vi "PAC-SLI.vi"() -> ()   [LabVIEW 2017]
uses:
  <vilib>/MakerHub/LINX/Private/Type Defs/Peripherals/SPI/SPI Configuration.ctl
  <vilib>/MakerHub/LINX/Private/Type Defs/Peripherals/SPI/SPI Bit Order.ctl
  <vilib>/MakerHub/LINX/Private/Type Defs/Peripherals/SPI/SPI Mode.ctl
  <vilib>/MakerHub/LINX/Public/Peripherals/SPI/SPI CS Config.ctl
  <vilib>/MakerHub/LINX/Private/Type Defs/Peripherals/SPI/SPI CS Logic Level.ctl
  <vilib>/Analysis/Matrix/Datatypes/RealMatrix.ctl
  <vilib>/MakerHub/LINX/Public/Peripherals/PWM/PWM Set Duty Cycle 1 Chan.vi
  <vilib>/MakerHub/LINX/Public/Peripherals/Analog/Analog Read 1 Chan.vi
  <vilib>/MakerHub/LINX/Public/Peripherals/Analog/Analog Read N Chans.vi
  <vilib>/MakerHub/LINX/Private/Local IO/LinxAnalogRead.vi
  <vilib>/MakerHub/LINX/Public/Utilities/Check Channel.vi
  <vilib>/MakerHub/LINX/Public/Utilities/Open Serial.vi
  <vilib>/MakerHub/LINX/Public/Peripherals/PWM/PWM Set Duty Cycle N Chans.vi
  <vilib>/MakerHub/LINX/Private/Utilties/Generate Error.vi
  <vilib>/Analysis/Matrix/Numeric/Conversions/Matrix To Array - RM.vi
  <vilib>/MakerHub/LINX/LMH-LINX.lvlib
  <vilib>/Analysis/Matrix/NI_Matrix.lvlib
panel:
  out "stop 2":bool
  out "Connection Initialized":bool
  out "Debug console":string
  in  "reset":bool
  in  "stop":bool
  out "I/O Device Name":string
  in  "?":T1(tab)
  in  "StayON 6":bool
  in  "StayON 5":bool
  in  "StayON 4":bool
  in  "StayON 3":bool
  in  "StayON 2":bool
  in  "StayON 1":bool
  in  "START Button":bool
  in  "Detector  6":bool
  out "Det 6 status":bool
  in  "Detector  5":bool
  out "Det 5 status":bool
  in  "Detector  4":bool
  out "Det 4 status":bool
  in  "Detector 3":bool
  out "Det 3 status":bool
  in  "Detector 2":bool
  out "Det 2 status":bool
  in  "Detector 1":bool
  out "Det 1 status":bool
  out "Photogate AIN":u8
  out "Stepper PUL DOUT":u8
  out "Stepper DIR DOUT":u8
  out "Stepper ENA DOUT":u8
  out "DigiPAC UART":u8
  out "Thermocouple 1":string
  out "Thermocouple 2":string
  out "Furnace ctrl Channel":u8
  out "Beam gate channel":u8
  in  "Furnace power% set":u8 max=100
  out "Furnace power%":u8
  out "Elapsed Super\nCycle Time (s)":dbl caption="Elapsed Time (s)"
  in  "Supercycle time [s]":dbl
  in  "CS Configuration":T2={"CS Channel"=7, "CS Logic Level"=enum."Active High"}
  in  "SPI Configuration":T4={"Clock Frequency"=1000000, "Bit Order"=enum."LSb First", "SPI Mode"=enum."Mode 0"}
  out "Clock Frequency":u32
  in  "CS Configuration 2":T2={"CS Channel"=7, "CS Logic Level"=enum."Active High"}
  in  "Photogate AIN":u8
  in  "Stepper PUL DOUT":u8
  in  "Stepper DIR DOUT":u8
  in  "Stepper ENA DOUT":u8
  in  "DigiPAC UART":u8
  in  "Furnace ctrl Channel":u8
  in  "Beam gate channel":u8
  in  "Operation|Time":T7
  in  "Serial Port":refnum<visa-resource-name>="COM3"
  # "Check settings before running!"
  # "I/O Channels"
  # "Temperature"
  # "Set      Status"
  # "Furnace power output"
  # "DIN.............."
  # "Digital input"
  # "DOUT.........."
  # "Digital output"
  # "AIN.............."
  # "Analog input"
  # "UART..........."
  # "Serial port"
  # "I/O ports"
  # "Thermocouple SPI settings"
  # "Automation order and timing"
  # "Thermocouple SPI settings required by MAX31855 amplifier:\nCS Logic level.............Active Low\nBit Order......................MSb First\nSPI Mode.....................Mode 0\nClock Frequency........<15000000\n                                      12500 is ok\nMISO/Data port...........50\nCLK port.......................52"
  # "Operation command numbers\n0, No action\n1, Detector acq. ON\n2, Detector acq. OFF\n3, Furnace power set\n4, Beam gate OFF\n5, Beam gate ON\n6, Furnace position IN\n7, Furnace position OUT\n8, Detector status check"
  # "Author: Mikko Kivekäs\nVersion: 0.2.0\nDate: 07/2019\nLicense: GPLv3\n\nThis program is created for PAC-SLI measurement setup in ISOLDE, CERN. This program is created for research use and should not be used in commercial applications.\n\nThis program is designed to be operated with Arduino Mega2560 I/O-board.  Communication between Arduino and this LabVIEW program uses serial communication over USB. MakerHub LINX library is used. https://www.labviewmakerhub.com/doku.php?id=libraries:linx:start\n\n\nIn monitoring tab user can monitor input and output values. Monitoring tab has also the control of detector data acquisition control. \n\nSettings tab contains all essential settings for running the measurement automation. There user can control I/O-ports, SPI settings and automation operation order and timing. SPI is used to read temperature values from MAX31855KASA+ thermocouple amplifier-adc. SPI MISO and CLK ports are fixed due Arduino design and stated under SPI-settings.\n\n     I/O type.....................I/O-port\n     -MISO/DO/Data.......50\n     -CLK/Clock...............52\n\nFurnace power setting I/O-port must be digital I/O-port with PMW. Choose of digital ports 2-13 (Arduino Mega2560). \n\nIndicator next to device name is ON when link between PC and Arduino is established and ready to run. Spress Start-button to run.\n\nCAUTION! FURNACE MUST BE IN UP POSITION, OTHERWISE FURNACE WILL BREAK DURING RUN.\n\nIf program does not run normally or you press \"Abort Execution\" of LabVIEW, build firmware to Arduino again. It is good practice to build firmware before\nevery run start. One can build firmware in LabVIEW going \n\n    Tools >> MakerHUB >> LINX >> LINX Firmware Wizard...  \n\nand there choosing right I/O-board and communication channel. In case of firmware not installing properly, disconnect all wires from Arduino, go to Arduino \nIDE and build in empty Sketch. If that does uploads properly, you can proceed to build LINX firmware.\n\nYou can find VIs and other information from https://github.com/MikkoKivekas/PAC-SLI"
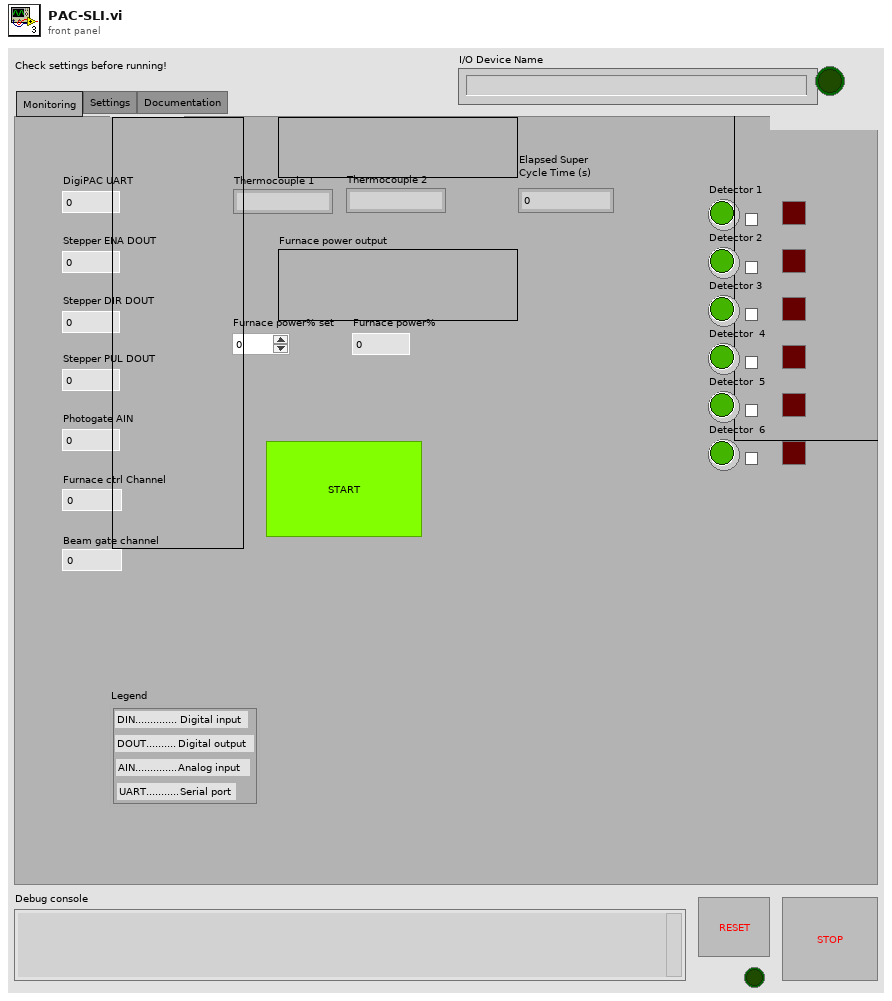
[diagram p1: front panel]
types:
  T1 = enum32{"Monitoring", "Settings", "Documentation"}
  T2 = typedef "LMH-LINX.lvlib/SPI CS Config.ctl" = cluster{"CS Channel":u8, "CS Logic Level":T3}
  T3 = typedef "LMH-LINX.lvlib/SPI CS Logic Level.ctl" = enum8{"Active Low", "Active High"}
  T4 = typedef "LMH-LINX.lvlib/SPI Configuration.ctl" = cluster{"Clock Frequency":u32, "Bit Order":T5, "SPI Mode":T6}
  T5 = typedef "LMH-LINX.lvlib/SPI Bit Order.ctl" = enum8{"LSb First", "MSb First"}
  T6 = typedef "LMH-LINX.lvlib/SPI Mode.ctl" = enum8{"Mode 0", "Mode 1", "Mode 2", "Mode 3"}
  T7 = typedef "NI_Matrix.lvlib/RealMatrix.ctl" = dbl[][]
  T8 = typedef "LMH-LINX.lvlib/LINX Ref.ctl" = cluster{"IO":T9, "Interface":T10, "LINX Device Config":T11}
  T9 = typedef "LMH-LINX.lvlib/Platform.ctl" = enum16{"Remote", "Local"}
  T10 = typedef "LMH-LINX.lvlib/Interface.ctl" = enum16{"Serial", "TCP"}
  T11 = typedef "LMH-LINX.lvlib/Device.lvlib/LINX Device Config.ctl" = cluster{"Interface":T10, "COM Port":refnum<visa-resource-name>, "TCP Configuration":T12, "Device Family":u8, "Device ID":u8, "Device Name":string, "TCP Ref":refnum<k5>, "Channels":T13}
  T12 = typedef "LMH-LINX.lvlib/Device.lvlib/TCP Config.ctl" = cluster{"IP Address":string, "Port":u16}
  T13 = typedef "LMH-LINX.lvlib/Channels.ctl" = cluster{"DI":u8[], "DO":u8[], "AI":u8[], "AO":u8[], "PWM":u8[], "QE":u8[], "UART":u8[], "I2C 2":u8[], "SPI":u8[], "CAN":u8[], "Servo":u8[], "AI Ref (V)":dbl, "AI Resolution (Bits)":u8, "AO Ref (V)":dbl, "AO Resolution (Bits)":u8}
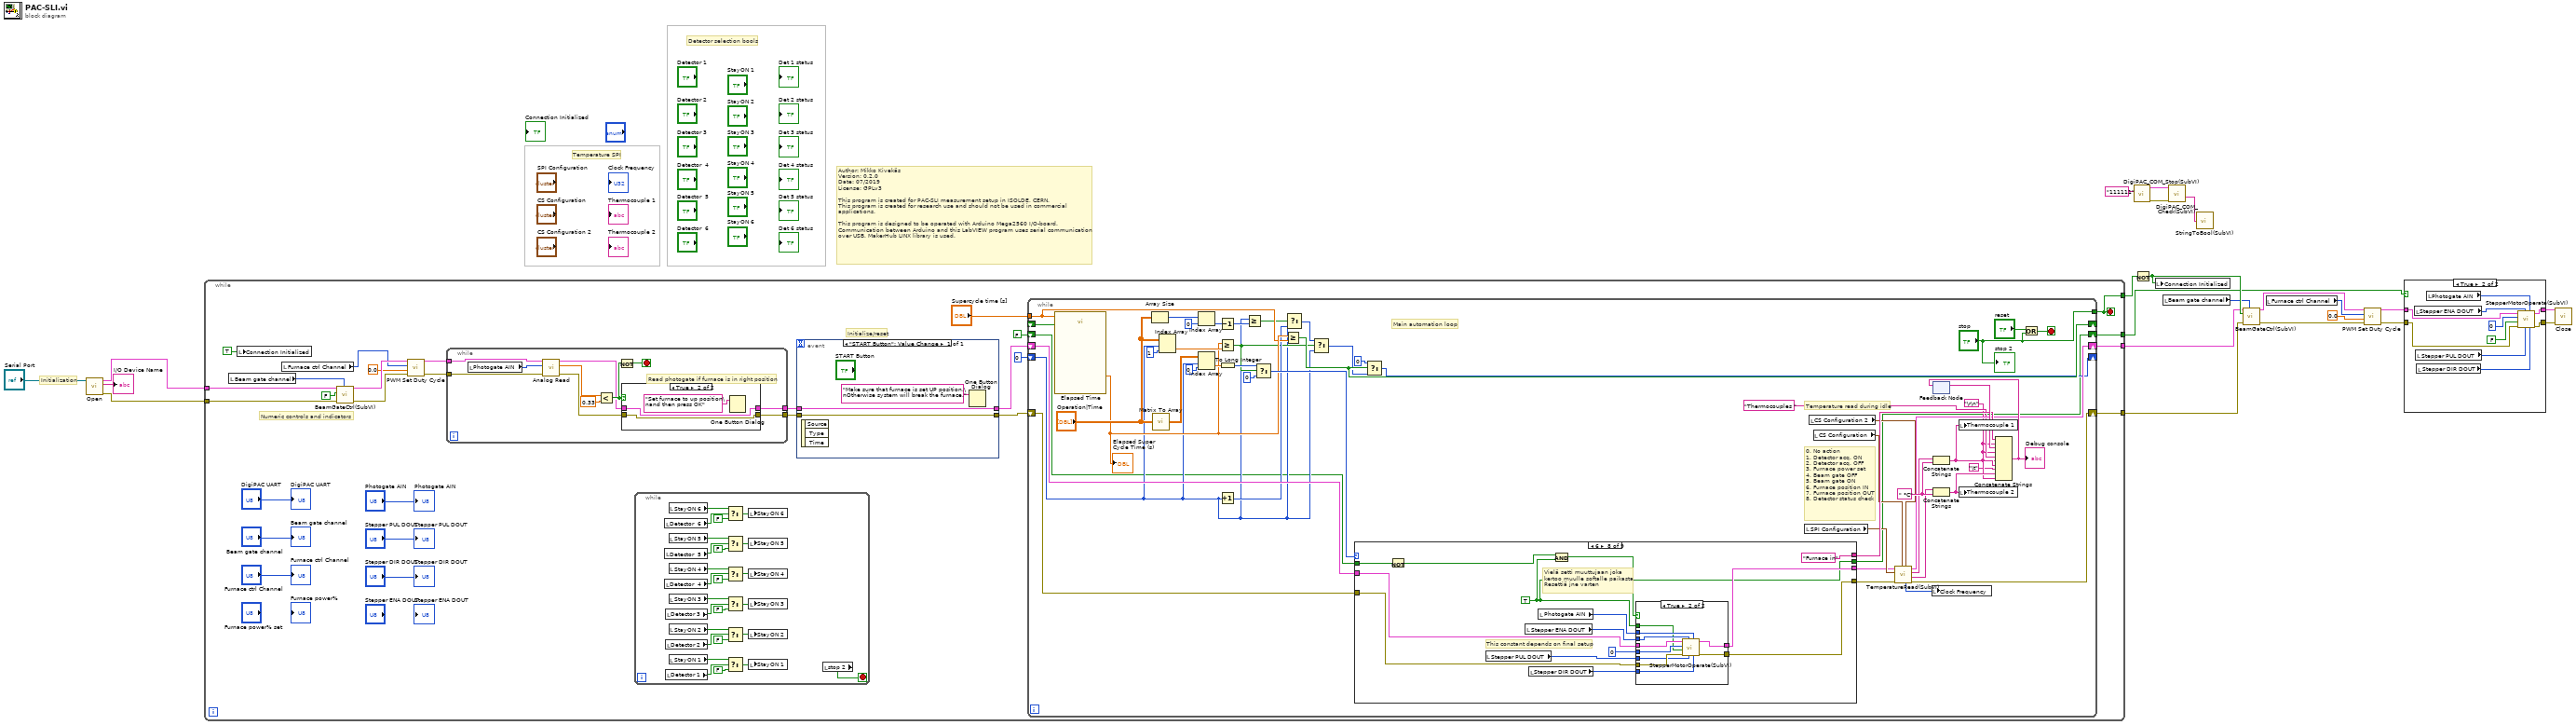
[diagram p0: block diagram]
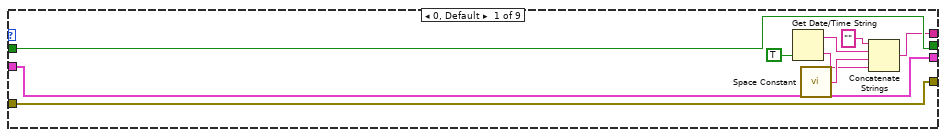
[diagram p4: hidden frame]
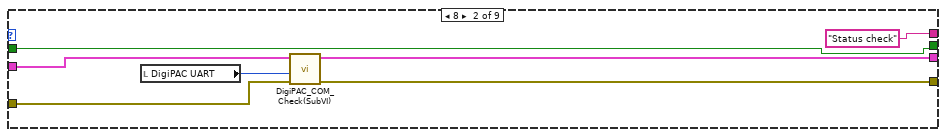
[diagram p5: hidden frame]
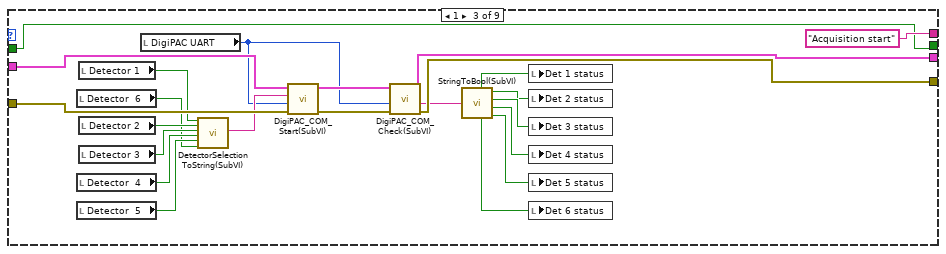
[diagram p6: hidden frame]
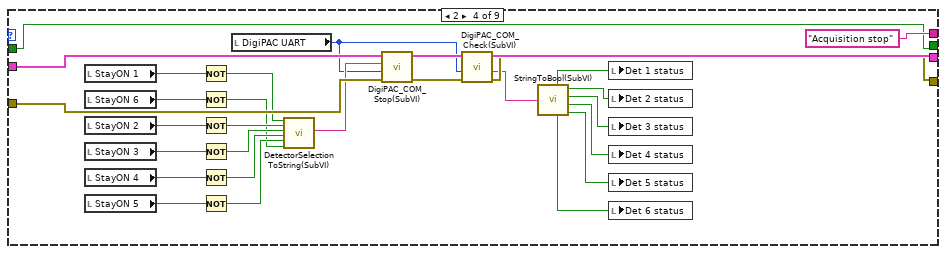
[diagram p7: hidden frame]
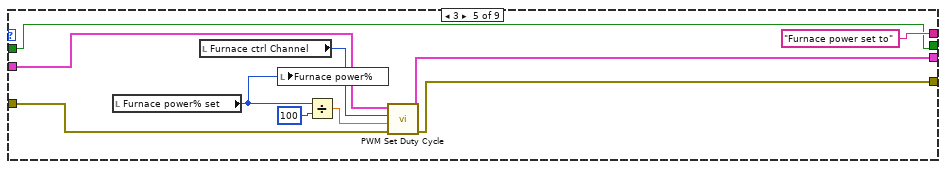
[diagram p8: hidden frame]
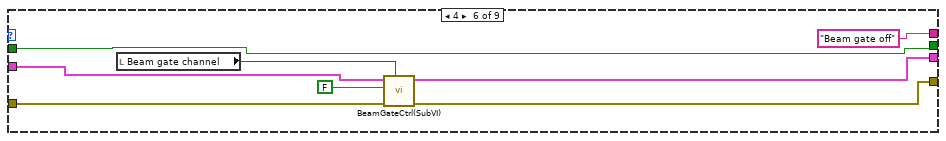
[diagram p9: hidden frame]
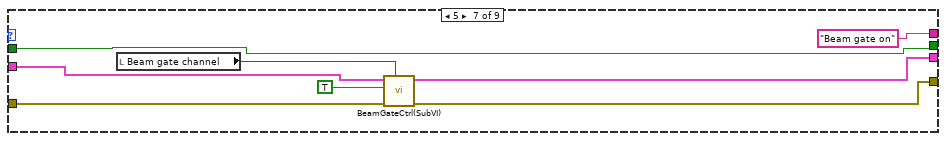
[diagram p10: hidden frame]
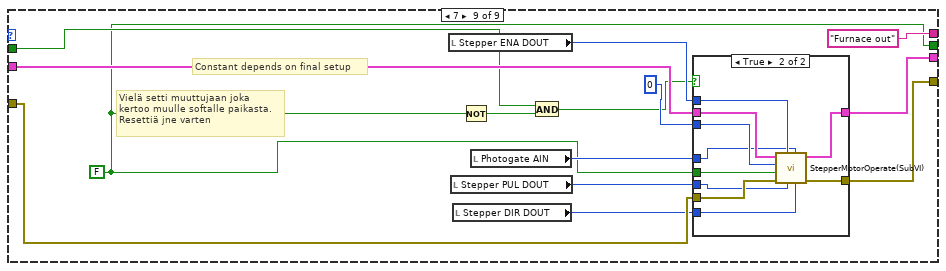
[diagram p12: hidden frame]
diagram:
  # "Author: Mikko Kivekäs\nVersion: 0.2.0\nDate: 07/2019\nLicense: GPLv3\n\nThis program is created for PAC-SLI measurement setup in ISOLDE, CERN.\nThis program is created for research use and should not be used in commercial\napplications.\n\nThis program is designed to be operated with Arduino Mega2560 I/O-board. \nCommunication between Arduino and this LabVIEW program uses serial communication\nover USB. MakerHub LINX library is used."
  # "Initialization"
  # "Temperature SPI"
  # "Detector selection bools"
  n1 = call-poly <vilib>:"Open.vi"("Serial Port"="Serial Port") -> ("Error Out"=w19:errorcluster, "Device Name"=→"I/O Device Name":string, "LINX Resource"=w20:T8)  [unwired: 8 in]
  n2 = while {
    tunnel: w20 -> [w35]
    tunnel: w19 -> [w34]
    tunnel: [w49] -> w15
    tunnel: [w48] -> w14
    tunnel: [w29] -> w18
    tunnel: [w43] -> w5
    stop <- w29 stop-if-true
    # "Numeric controls and indicators"
    # "Initialize/reset"
    n3 = local read "Beam gate channel"() -> (w30:u8)
    n4 = local write "Connection Initialized"(TRUE ("Connection Initialized")) -> ()
    n5 = local read "Furnace ctrl Channel"() -> (w31:u8)
    n6 = call "BeamGateCtrl(SubVI).vi"("Beam gate ctrl channel"=w30, "Error In"=w34, "Output Value"=FALSE, "LINX Resource"=w35) -> ("Error Out"=w38:errorcluster, "LINX Resource 2"=w39:T8)  [unwired: 6 in]
    n7 = call-poly <vilib>:"PWM Set Duty Cycle.vi"("Error In"=w38, "Duty Cycle (0-1)"=0.0, "PWM Channel"=w31, "LINX Resource"=w39) -> ("Error Out"=w36:errorcluster, "LINX Resource"=w37:T8)  [unwired: 6 in]
    n8 = while {
      tunnel: w37 -> [w81]
      tunnel: [w79] -> w41
      tunnel: w36 -> [w78]
      tunnel: [w76] -> w40
      stop <- w82 stop-if-true
      # "Read photogate if furnace is in right position"
      n9 = local read "Photogate AIN"() -> (w84:u8)
      n10 = call-poly <vilib>:"Analog Read.vi"("Error In"=w78, "Analog Channel"=w84, "LINX Resource"=w81) -> ("Error Out"=w77:errorcluster, "Voltage"=w86:dbl, "LINX Resource"=w80:T8)  [unwired: 5 in, 1 out]
      n11 = Less?(x=w86, y=0.33) -> (x < y?=w83:bool)
      n12 = Not(x=w83) -> (.not. x?=w82:bool)
      n13 = case shown="True" w83 {
        tunnel: w80 -> [w88 w90]
        tunnel: [w88 w90] -> w79
        tunnel: w77 -> [w87 w89]
        tunnel: [w87 w89] -> w76
        frame False {
        }
        frame True {
          n14 = One Button Dialog(message="Set furnace to up position\nand then press OK") -> ()  [unwired: 1 in, 1 out]
        }
      }
    }
    n15 = while {
      stop <- w51 stop-if-true
      n16 = local read "Detector  6"() -> (w74:bool)
      n17 = local read "Detector  5"() -> (w72:bool)
      n18 = local read "Detector  4"() -> (w70:bool)
      n19 = local read "Detector 3"() -> (w68:bool)
      n20 = local read "Detector 2"() -> (w66:bool)
      n21 = local read "Detector 1"() -> (w64:bool)
      n22 = local read "StayON 6"() -> (w75:bool)
      n23 = local read "StayON 5"() -> (w73:bool)
      n24 = local read "StayON 4"() -> (w71:bool)
      n25 = local read "StayON 3"() -> (w69:bool)
      n26 = local read "StayON 2"() -> (w67:bool)
      n27 = local read "StayON 1"() -> (w65:bool)
      n28 = Select(t=w75, s=w74, f=FALSE) -> (s? t:f=w63:bool)
      n29 = Select(t=w73, s=w72, f=FALSE) -> (s? t:f=w62:bool)
      n30 = Select(t=w71, s=w70, f=FALSE) -> (s? t:f=w61:bool)
      n31 = Select(t=w69, s=w68, f=FALSE) -> (s? t:f=w60:bool)
      n32 = Select(t=w67, s=w66, f=FALSE) -> (s? t:f=w59:bool)
      n33 = Select(t=w65, s=w64, f=FALSE) -> (s? t:f=w58:bool)
      n34 = local write "StayON 6"(w63) -> ()
      n35 = local write "StayON 5"(w62) -> ()
      n36 = local write "StayON 4"(w61) -> ()
      n37 = local write "StayON 3"(w60) -> ()
      n38 = local write "StayON 2"(w59) -> ()
      n39 = local write "StayON 1"(w58) -> ()
      n40 = local read "stop 2"() -> (w51:bool)
    }
    n41 = event shown="[0] \"START Button\": Value Change" {
      selector: _ -> [_]
      dyn-events: _ -> [_]
      timeout: _ -> [_]
      tunnel: w41 -> [w93]
      tunnel: [w93] -> w46
      tunnel: w40 -> [w92]
      tunnel: [w92] -> w45
      event "START Button": Value Change {
        n42 = event-data() -> ()  [unwired: 1 in, 3 out]
        n43 = One Button Dialog(message="Make sure that furnace is set UP position.\nOtherwise system will break the furnace.") -> ()  [unwired: 1 in, 1 out]
      }
    }
    n44 = while {
      tunnel: ["stop"] -> w29
      shift-right: [w98] -> _
      shift-left: 0 -> [w97]
      shift-right: [w125] -> w49
      shift-left: w46 -> [w142]
      shift-right: [w124] -> w48
      shift-left: w45 -> [w141]
      tunnel: "Supercycle time [s]" -> [w107]
      shift-right: [w105] -> _
      shift-left: _ -> [w106]
      shift-right: [w96] -> w43
      shift-left: FALSE ("Direction input") -> [w95]
      stop <- w145 stop-if-true
      w110 = "\r\n"
      w136 = " °C"
      # "0, No action\n1, Detector acq. ON\n2, Detector acq. OFF\n3, Furnace power set\n4, Beam gate OFF\n5, Beam gate ON\n6, Furnace position IN\n7, Furnace position OUT\n8, Detector status check"
      # "Temperature read during idle"
      # "Main automation loop"
      n45 = call "Elapsed Time"("Time Target (s)"=w107, "Reset"=w106) -> ("Elapsed Time (s)"=w108:dbl)  [unwired: 10 in, 7 out]
      "Elapsed Super\nCycle Time (s)" <- w108
      n46 = Array Size(array="Operation|Time") -> (size(s)=w140:i32[])
      n47 = call-poly <vilib>:"Matrix To Array.vi"("Real Matrix"="Operation|Time") -> ("Real 2D Array"=w138:dbl[][])
      n48 = Index Array(array="Operation|Time", index (row)=w97, index (col)=1 ("disabled index (col)")) -> (element=w117:dbl)
      n49 = Index Array(array=w140, index=0) -> (element=w133:i32)
      n50 = Index Array(array=w138, index (row)=w97, index (col)=0 ("disabled index (col)")) -> (element=w135:dbl)
      n51 = Decrement(x=w133) -> (x-1=w134:i32)
      n52 = Greater Or Equal?(x=w108, y=w117) -> (x >= y?=w100:bool)
      n53 = To Long Integer(number=w135) -> (32bit integer=w116:i32)
      n54 = Increment(x=w97) -> (x+1=w103:i32)
      n55 = Greater Or Equal?(x=w97, y=w134) -> (x >= y?=w102:bool)
      n56 = Select(t=w116, s=w100, f=0) -> (s? t:f=w114:i32)
      n57 = Greater Or Equal?(x=w108, y=w107) -> (x >= y?=w105:bool)
      n58 = Select(t=w97, s=w102, f=w103) -> (s? t:f=w101:i32)
      n59 = Select(t=w101, s=w100, f=w97) -> (s? t:f=w99:i32)
      n60 = case shown="6" w114 {
        tunnel: w142 -> [w154 w160 w184 w213 w223 w231 w239 w253 w279]
        tunnel: [w154 w159 w182 w211 w222 w228 w236 w252 w278] -> w127
        tunnel: w141 -> [w153 w158 w181 w208 w221 w229 w237 w250 w276]
        tunnel: [w153 w157 w179 w210 w220 w227 w235 w251 w277] -> w126
        tunnel: [w149 "Status check" "Acquisition start" "Acquisition stop" "Furnace power set to" "Beam gate off" "Beam gate on" "Furnace in" "Furnace out"] -> w130
        tunnel: [w152 w155 w162 w185 w217 w224 w232 w241 w267] -> w96
        tunnel: w95 -> [w152 w155 w162 w185 w217 w224 w232 w242 w268]
        frame 0, Default {
          n61 = Get Date/Time String(want seconds? (F)=TRUE) -> (date string=w151:string, time string=w146:string)  [unwired: 2 in]
          n62 = call <vilib>:"Space Constant.vi"() -> ("String"=w147:string)
          n63 = Concatenate Strings("", w151, w147, w146) -> (w149:string)
        }
        frame 8 {
          n64 = local read "DigiPAC UART"() -> (w156:u8)
          n65 = call "DigiPAC_COM_Check(SubVI).vi"("error in (no error)"=w158, "UART Channel (0)"=w156, "LINX Resource in"=w160) -> ("error out"=w157:errorcluster, "LINX Resource out"=w159:T8)  [unwired: 5 in, 2 out]
        }
        frame 1 {
          n66 = local read "Detector  6"() -> (w165:bool)
          n67 = local read "Detector  4"() -> (w167:bool)
          n68 = local read "Detector  5"() -> (w166:bool)
          n69 = local read "Detector 1"() -> (w170:bool)
          n70 = local read "Detector 2"() -> (w169:bool)
          n71 = local read "Detector 3"() -> (w168:bool)
          n72 = local read "DigiPAC UART"() -> (w164:u8)
          n73 = call "DetectorSelectionToString(SubVI).vi"("Detector 1"=w170, "Detector 2"=w169, "Detector 3"=w168, "Detector 4"=w167, "Detector 5"=w166, "Detector 6"=w165) -> ("Output strting"=w171:string)  [unwired: 13 in]
          n74 = call "DigiPAC_COM_Start(SubVI).vi"("error in (no error)"=w181, "UART Channel (0)"=w164, "Detector input"=w171, "LINX Resource in"=w184) -> ("error out"=w180:errorcluster, "LINX Resource out"=w183:T8)  [unwired: 5 in, 1 out]
          n75 = call "DigiPAC_COM_Check(SubVI).vi"("error in (no error)"=w180, "UART Channel (0)"=w164, "LINX Resource in"=w183) -> ("error out"=w179:errorcluster, "Confirmation message"=w178:string, "LINX Resource out"=w182:T8)  [unwired: 5 in, 1 out]
          n76 = call "StringToBool(SubVI).vi"("string"=w178) -> ("Det 1"=w172:bool, "Det 2"=w173:bool, "Det 3"=w174:bool, "Det 6"=w177:bool, "Det 4"=w175:bool, "Det 5"=w176:bool)  [unwired: 4 in]
          n77 = local write "Det 1 status"(w172) -> ()
          n78 = local write "Det 2 status"(w173) -> ()
          n79 = local write "Det 3 status"(w174) -> ()
          n80 = local write "Det 4 status"(w175) -> ()
          n81 = local write "Det 5 status"(w176) -> ()
          n82 = local write "Det 6 status"(w177) -> ()
        }
        frame 2 {
          n83 = local read "StayON 1"() -> (w200:bool)
          n84 = local read "StayON 6"() -> (w195:bool)
          n85 = local read "StayON 2"() -> (w199:bool)
          n86 = local read "StayON 3"() -> (w198:bool)
          n87 = local read "StayON 4"() -> (w197:bool)
          n88 = local read "StayON 5"() -> (w196:bool)
          n89 = Not(x=w200) -> (.not. x?=w206:bool)
          n90 = Not(x=w195) -> (.not. x?=w201:bool)
          n91 = Not(x=w199) -> (.not. x?=w205:bool)
          n92 = Not(x=w198) -> (.not. x?=w204:bool)
          n93 = Not(x=w197) -> (.not. x?=w203:bool)
          n94 = Not(x=w196) -> (.not. x?=w202:bool)
          n95 = local read "DigiPAC UART"() -> (w193:u8)
          n96 = call "DetectorSelectionToString(SubVI).vi"("Detector 1"=w206, "Detector 2"=w205, "Detector 3"=w204, "Detector 4"=w203, "Detector 5"=w202, "Detector 6"=w201) -> ("Output strting"=w207:string)  [unwired: 13 in]
          n97 = call "DigiPAC_COM_Stop(SubVI).vi"("error in (no error)"=w208, "UART Channel (0)"=w193, "Detector input"=w207, "LINX Resource in"=w213) -> ("error out"=w209:errorcluster, "LINX Resource out"=w212:T8)  [unwired: 5 in, 1 out]
          n98 = call "DigiPAC_COM_Check(SubVI).vi"("error in (no error)"=w209, "UART Channel (0)"=w193, "LINX Resource in"=w212) -> ("error out"=w210:errorcluster, "Confirmation message"=w194:string, "LINX Resource out"=w211:T8)  [unwired: 5 in, 1 out]
          n99 = call "StringToBool(SubVI).vi"("string"=w194) -> ("Det 1"=w187:bool, "Det 2"=w188:bool, "Det 3"=w189:bool, "Det 6"=w192:bool, "Det 4"=w190:bool, "Det 5"=w191:bool)  [unwired: 4 in]
          n100 = local write "Det 1 status"(w187) -> ()
          n101 = local write "Det 2 status"(w188) -> ()
          n102 = local write "Det 3 status"(w189) -> ()
          n103 = local write "Det 4 status"(w190) -> ()
          n104 = local write "Det 5 status"(w191) -> ()
          n105 = local write "Det 6 status"(w192) -> ()
        }
        frame 3 {
          n106 = local read "Furnace power% set"() -> (w214:u8)
          n107 = local read "Furnace ctrl Channel"() -> (w219:u8)
          n108 = local write "Furnace power%"(w214) -> ()
          n109 = Divide(x=w214, y=u8 100) -> (x/y=w216:dbl)
          n110 = call-poly <vilib>:"PWM Set Duty Cycle.vi"("Error In"=w221, "Duty Cycle (0-1)"=w216, "PWM Channel"=w219, "LINX Resource"=w223) -> ("Error Out"=w220:errorcluster, "LINX Resource"=w222:T8)  [unwired: 6 in]
        }
        frame 4 {
          n111 = local read "Beam gate channel"() -> (w230:u8)
          n112 = call "BeamGateCtrl(SubVI).vi"("Beam gate ctrl channel"=w230, "Error In"=w229, "Output Value"=FALSE, "LINX Resource"=w231) -> ("Error Out"=w227:errorcluster, "LINX Resource 2"=w228:T8)  [unwired: 6 in]
        }
        frame 5 {
          n113 = local read "Beam gate channel"() -> (w238:u8)
          n114 = call "BeamGateCtrl(SubVI).vi"("Beam gate ctrl channel"=w238, "Error In"=w237, "Output Value"=TRUE, "LINX Resource"=w239) -> ("Error Out"=w235:errorcluster, "LINX Resource 2"=w236:T8)  [unwired: 6 in]
        }
        frame 6 {
          w241 = TRUE ("Direction input")
          # "Vielä setti muuttujaan joka \nkertoo muulle softalle paikasta.\nResettiä jne varten"
          # "This constant depends on final setup"
          n115 = Not(x=w242) -> (.not. x?=w243:bool)
          n116 = local read "Stepper PUL DOUT"() -> (w249:u8)
          n117 = local read "Stepper ENA DOUT"() -> (w246:u8)
          n118 = local read "Stepper DIR DOUT"() -> (w248:u8)
          n119 = local read "Photogate AIN"() -> (w245:u8)
          n120 = And(x=w243, y=w241) -> (x .and. y?=w240:bool)
          n121 = case shown="True" w240 {
            tunnel: w253 -> [w255 w265]
            tunnel: [w255 w264] -> w252
            tunnel: [w254 w263] -> w251
            tunnel: w250 -> [w254 w262]
            tunnel: w249 -> [_ w261]
            tunnel: w248 -> [_ w260]
            tunnel: 0 ("Maximum steps\ninput") -> [_ w259]
            tunnel: w246 -> [_ w258]
            tunnel: w245 -> [_ w257]
            tunnel: w241 -> [_ w256]
            frame False {
            }
            frame True {
              n122 = call "StepperMotorOperate(SubVI).vi"("DIR channel"=w260, "Photogate channel"=w257, "PUL channel"=w261, "ENA channel"=w258, "error in (no error)"=w262, "Direction input"=w256, "Maximum steps\ninput"=w259, "LINX Resource in"=w265) -> ("error out"=w263:errorcluster, "LINX Resource out"=w264:T8)  [unwired: 2 in]
            }
          }
        }
        frame 7 {
          w267 = FALSE ("Direction input")
          # "Vielä setti muuttujaan joka \nkertoo muulle softalle paikasta.\nResettiä jne varten"
          # "Constant depends on final setup"
          n123 = local read "Stepper ENA DOUT"() -> (w272:u8)
          n124 = local read "Stepper PUL DOUT"() -> (w275:u8)
          n125 = local read "Stepper DIR DOUT"() -> (w274:u8)
          n126 = Not(x=w267) -> (.not. x?=w269:bool)
          n127 = local read "Photogate AIN"() -> (w271:u8)
          n128 = And(x=w268, y=w269) -> (x .and. y?=w266:bool)
          n129 = case shown="True" w266 {
            tunnel: w279 -> [w281 w291]
            tunnel: [w281 w290] -> w278
            tunnel: [w280 w289] -> w277
            tunnel: w276 -> [w280 w288]
            tunnel: w275 -> [_ w287]
            tunnel: w274 -> [_ w286]
            tunnel: 0 ("Maximum steps\ninput") -> [_ w285]
            tunnel: w272 -> [_ w284]
            tunnel: w271 -> [_ w283]
            tunnel: w267 -> [_ w282]
            frame False {
            }
            frame True {
              n130 = call "StepperMotorOperate(SubVI).vi"("DIR channel"=w286, "Photogate channel"=w283, "PUL channel"=w287, "ENA channel"=w284, "error in (no error)"=w288, "Direction input"=w282, "Maximum steps\ninput"=w285, "LINX Resource in"=w291) -> ("error out"=w289:errorcluster, "LINX Resource out"=w290:T8)  [unwired: 2 in]
            }
          }
        }
      }
      n131 = Select(t=u8 0, s=w105, f=w99) -> (s? t:f=w98:i32)
      n132 = local read "SPI Configuration"() -> (w128:T4)
      n133 = local read "CS Configuration 2"() -> (w121:T2)
      n134 = local read "CS Configuration"() -> (w120:T2)
      n135 = call "TemperatureRead(SubVI).vi"("CS Configuration 2"=w121, "CS Configuration"=w120, "Error In"=w126, "SPI Configuration"=w128, "LINX Resource"=w127) -> ("Error Out"=w124:errorcluster, "Temp2"=w122:string, "Temp1"=w123:string, "LINX Resource 2"=w125:T8, "Actual Clock Frequency"=w129:u32)  [unwired: 2 in]
      n136 = local write "Clock Frequency"(w129) -> ()
      n137 = feedback #1() -> (w132:string)  [unwired: 1 in]
      n138 = Concatenate Strings(w123, w136) -> (w112:string)
      n139 = Concatenate Strings(w122, w136) -> (w111:string)
      n140 = local write "Thermocouple 1"(w112) -> ()
      n141 = local write "Thermocouple 2"(w111) -> ()
      n142 = Concatenate Strings(w130, w110, w132, w110, "Thermocouples ", w110, w112, "\t", w111, w110) -> (w131:string)
      "Debug console" <- w131
      n143 = feedback-in #1(w131) -> ()
      n144 = Or(x="reset", y="stop") -> (x .or. y?=w145:bool)
      "stop 2" <- "stop"
    }
    "DigiPAC UART" <- "DigiPAC UART"
    "Furnace ctrl Channel" <- "Furnace ctrl Channel"
    "Beam gate channel" <- "Beam gate channel"
    "Stepper DIR DOUT" <- "Stepper DIR DOUT"
    "Stepper PUL DOUT" <- "Stepper PUL DOUT"
    "Photogate AIN" <- "Photogate AIN"
  }
  n145 = call "DigiPAC_COM_Stop(SubVI).vi"("Detector input"="111111") -> ("error out"=w8:errorcluster, "LINX Resource out"=w9:T8)  [unwired: 8 in, 1 out]
  n146 = Not(x=w18) -> (.not. x?=w17:bool)
  n147 = local write "Connection Initialized"(w17) -> ()
  n148 = local read "Beam gate channel"() -> (w11:u8)
  n149 = call "DigiPAC_COM_Check(SubVI).vi"("error in (no error)"=w8, "LINX Resource in"=w9) -> ("Confirmation message"=w6:string)  [unwired: 6 in, 3 out]
  n150 = call "StringToBool(SubVI).vi"("string"=w6) -> ()  [unwired: 4 in, 6 out]
  n151 = call "BeamGateCtrl(SubVI).vi"("Beam gate ctrl channel"=w11, "Error In"=w14, "Output Value"=w17, "LINX Resource"=w15) -> ("Error Out"=w12:errorcluster, "LINX Resource 2"=w16:T8)  [unwired: 6 in]
  n152 = local read "Furnace ctrl Channel"() -> (w10:u8)
  n153 = call-poly <vilib>:"PWM Set Duty Cycle.vi"("Error In"=w12, "Duty Cycle (0-1)"=0.0, "PWM Channel"=w10, "LINX Resource"=w16) -> ("Error Out"=w3:errorcluster, "LINX Resource"=w4:T8)  [unwired: 6 in]
  n154 = case shown="True" w5 {
    tunnel: w4 -> [w293 w302]
    tunnel: w3 -> [w292 w303]
    tunnel: [w293 w301] -> w2
    tunnel: [w292 w300] -> w1
    frame False {
    }
    frame True {
      n155 = local read "Stepper ENA DOUT"() -> (w298:u8)
      n156 = local read "Stepper PUL DOUT"() -> (w295:u8)
      n157 = local read "Stepper DIR DOUT"() -> (w296:u8)
      n158 = local read "Photogate AIN"() -> (w297:u8)
      n159 = call "StepperMotorOperate(SubVI).vi"("DIR channel"=w296, "Photogate channel"=w297, "PUL channel"=w295, "ENA channel"=w298, "error in (no error)"=w303, "Direction input"=FALSE, "Maximum steps\ninput"=0 ("Maximum steps\ninput"), "LINX Resource in"=w302) -> ("error out"=w300:errorcluster, "LINX Resource out"=w301:T8)  [unwired: 2 in]
    }
  }
  n160 = call <vilib>:"Close.vi"("Error In"=w1, "LINX Resource"=w2) -> ()  [unwired: 9 in, 1 out]
